vi "TOP VI-aim lab.vi"() -> ()   [LabVIEW 2014]
uses:
  <vilib>/Utility/miscctls.llb/LVPoint32TypeDef.ctl
  <vilib>/Utility/miscctls.llb/LVPositionTypeDef.ctl
panel:
  out "RECORD":bool
  in  "player name":string="player 1"
  out "element":T1(ring)
  out "seconds":dbl
  out "millisecond timer value 2":u32
  out "millisecond timer value":u32
  out "finish ?":bool
  out "Boolean":bool
  out "hit coord":T2
  in  "aim":bool
  in  "normal":bool
  in  "number of targets":i32=10
  in  "spacing limit":i32=5
  out "records":string[][](table)
  in  "New Game":bool
  in  "Quit":bool
  out "Game Image":picture
  # "true for aim mode"
  # "user discription:\npress New Game before run ensure parameters was set.\nchose mode with the lowest button;\npractice mode doesnt get records;\naim mode get records;\nrecords renew when vi restart;\nset name and parameter up to the \ndiscription;\npress New Game to change the number of targets & spacing limit;\n\n註記：\n右邊的picture大小可能與電腦螢幕大小有關，可用property調整為該使用者適當的螢幕大小，若是無法跑動，把play aim set target 跟generate target這兩個sub vi的cluster array重新創一次(不知道為啥有時會跑掉。目標有可能出現在視窗邊邊，須留意，畢竟有時敵人也只有露半個頭。"
  # "user pane"
  # "game pane"
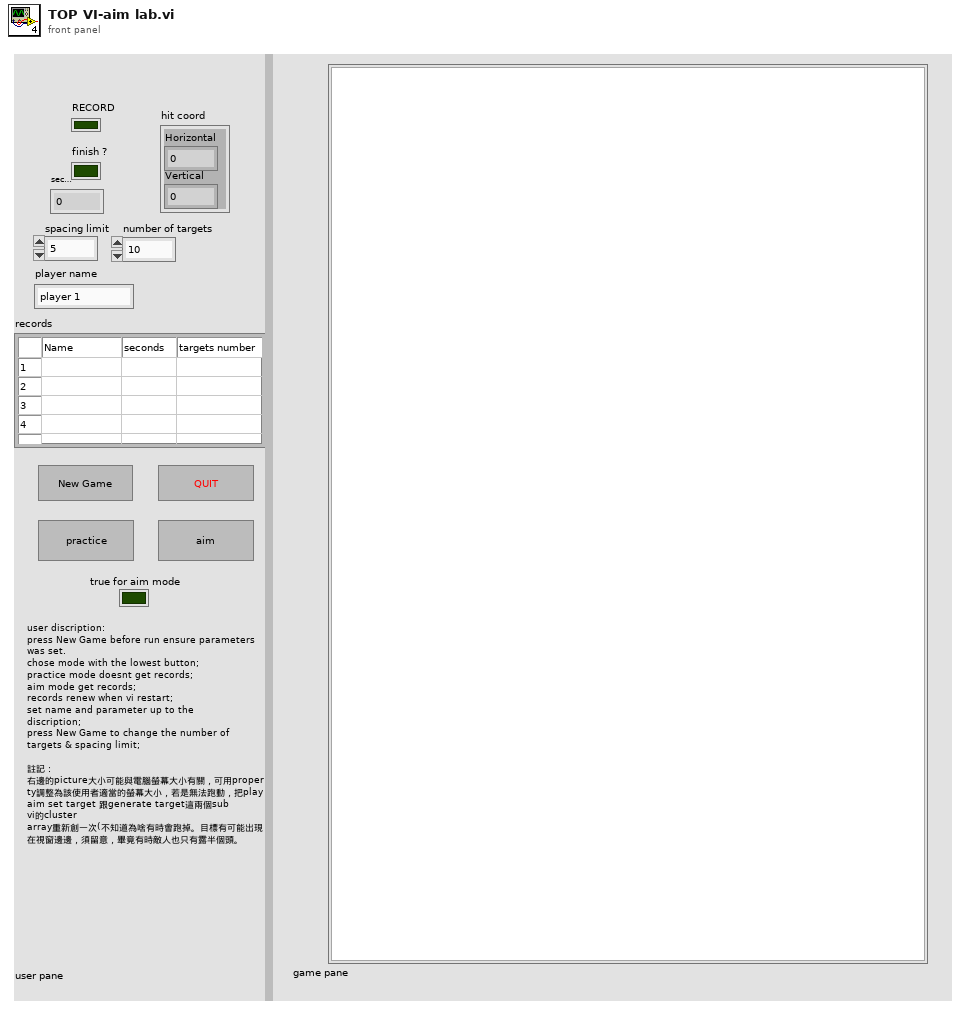
[diagram p1: front panel]
types:
  T1 = enum16{"waits function", "new game(reset)", "play normal", "play aim", "check hit", "quit", "draw target", "draw target for aim"}
  T2 = typedef "LVPoint32TypeDef.ctl" = cluster{"Horizontal":i32, "Vertical":i32}
  T3 = typedef "LVPositionTypeDef.ctl" = cluster{"Left":i32, "Top":i32}
  T4 = enum16{"nothing", "quit", "in play(normal or aim)"}
  T5 = enum16{"waits function", "new game(reset)", "play normal", "play aim", "check hit", "quit"}
  T6 = enum8{"Enabled", "Disabled", "Disabled and Grayed Out"}
  T7 = enum16{"waits function", "new game(reset)", "play normal", "play aim", "check hit", "quit", "draw target"}
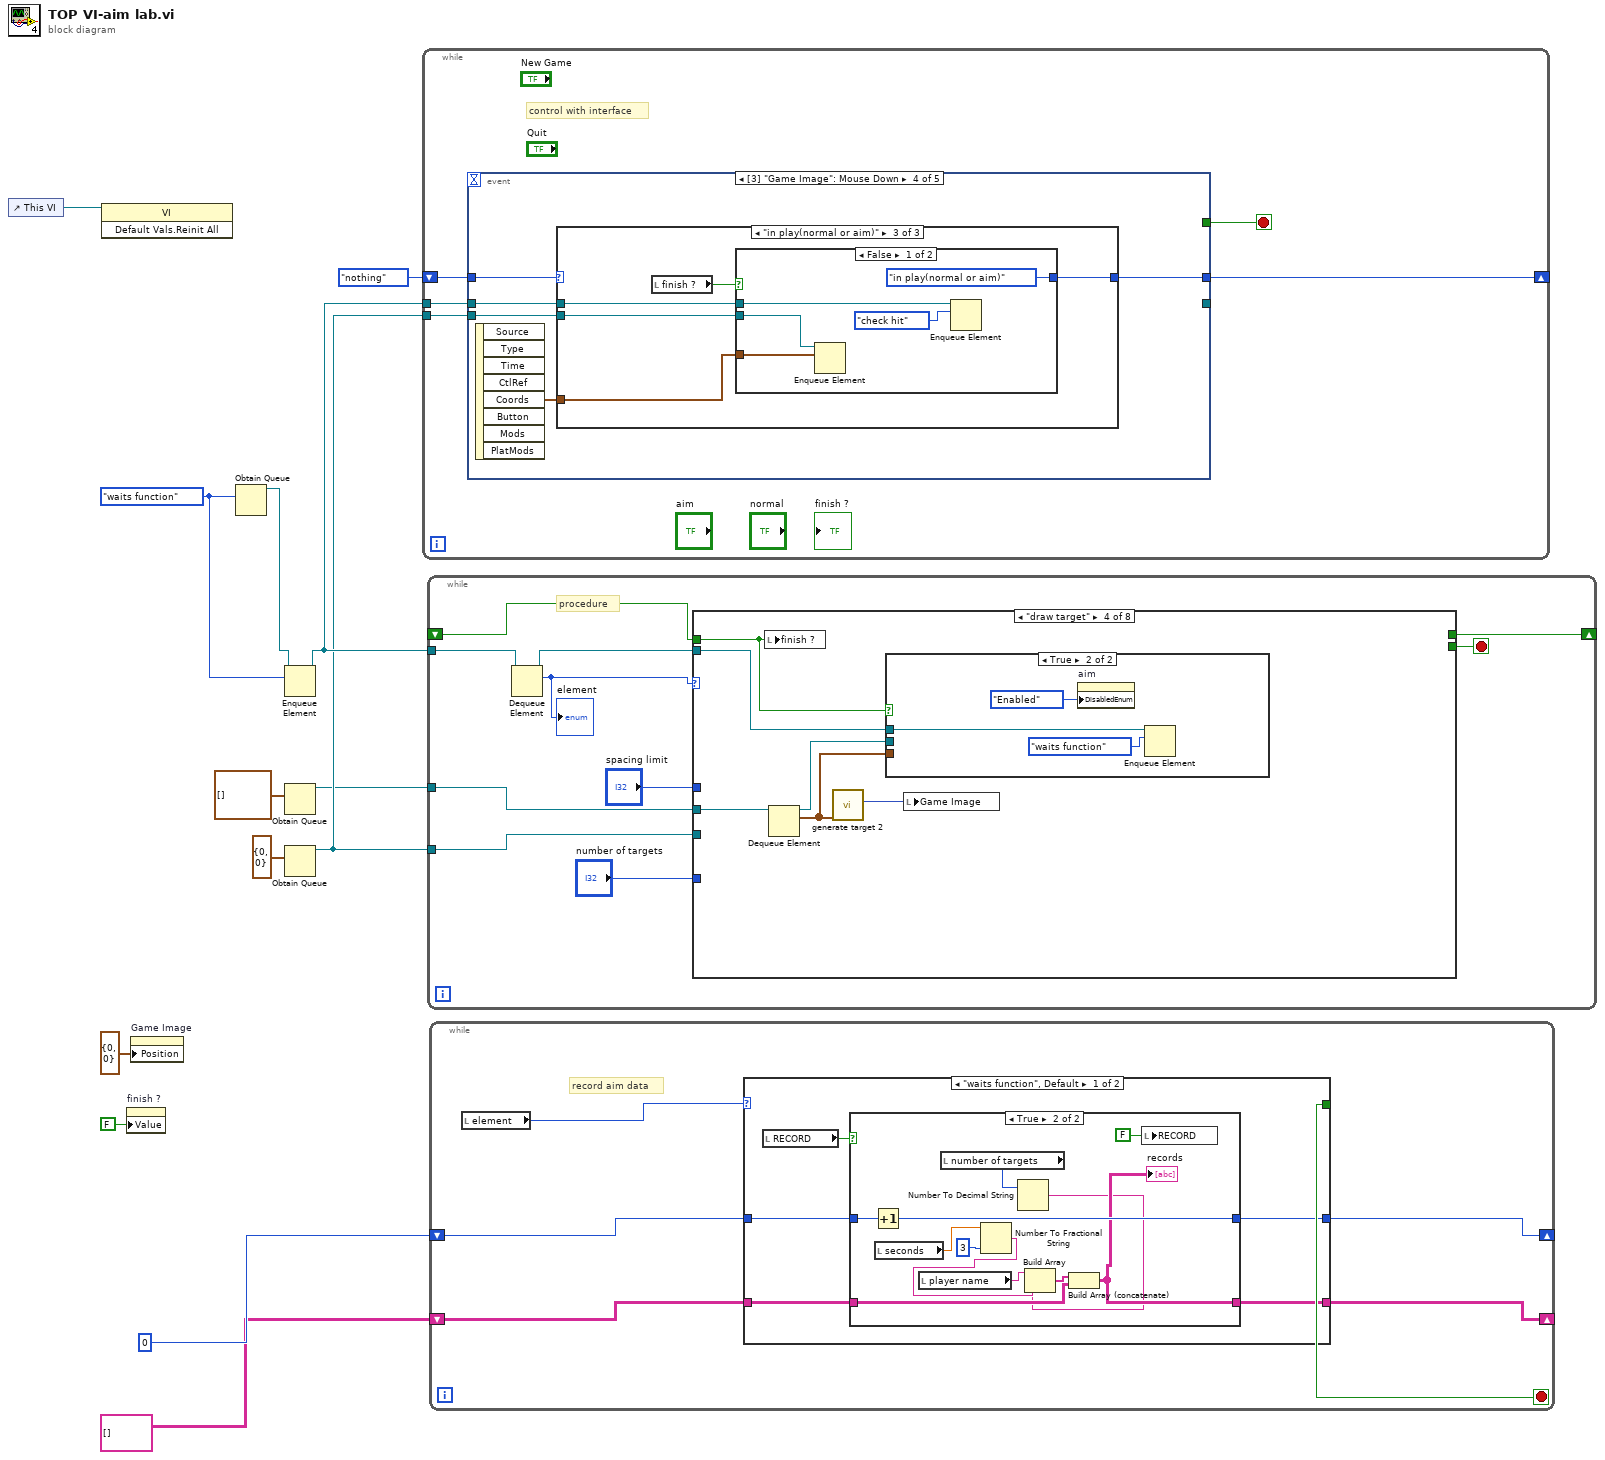
[diagram p0: block diagram]
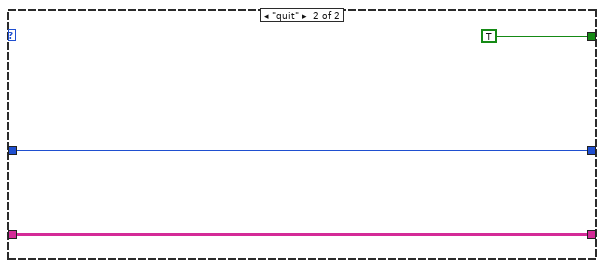
[diagram p3: hidden frame]
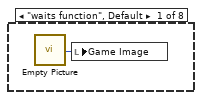
[diagram p4: hidden frame]
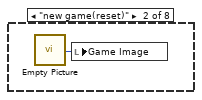
[diagram p5: hidden frame]
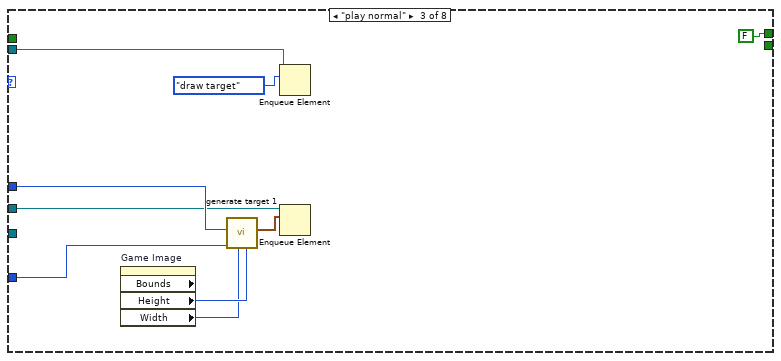
[diagram p6: hidden frame]
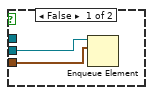
[diagram p7: hidden frame]
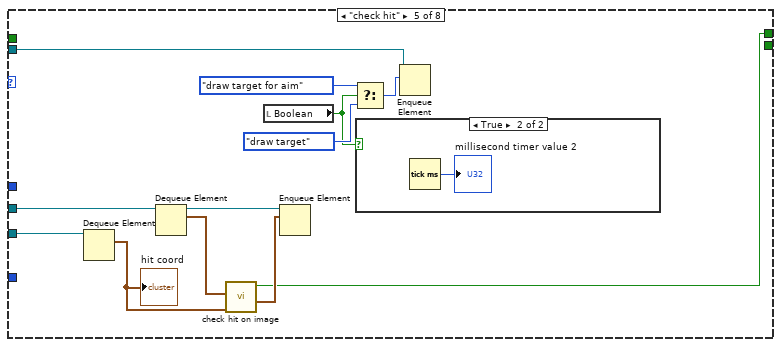
[diagram p8: hidden frame]
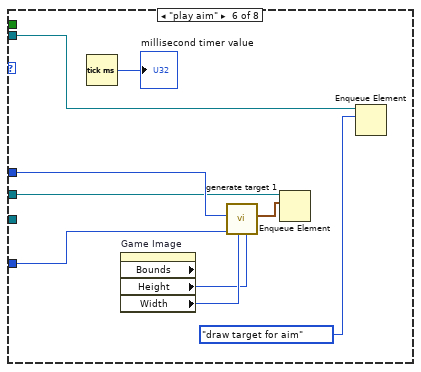
[diagram p10: hidden frame]
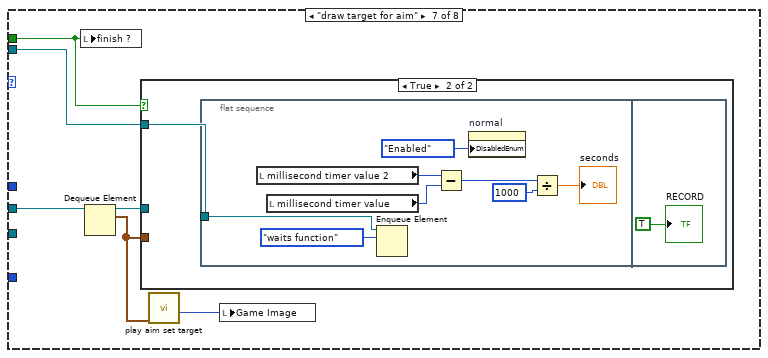
[diagram p11: hidden frame]
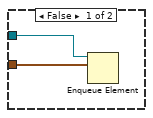
[diagram p12: hidden frame]
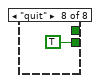
[diagram p13: hidden frame]
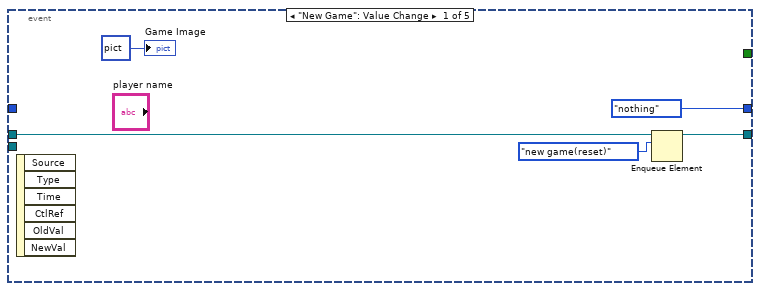
[diagram p14: hidden frame]
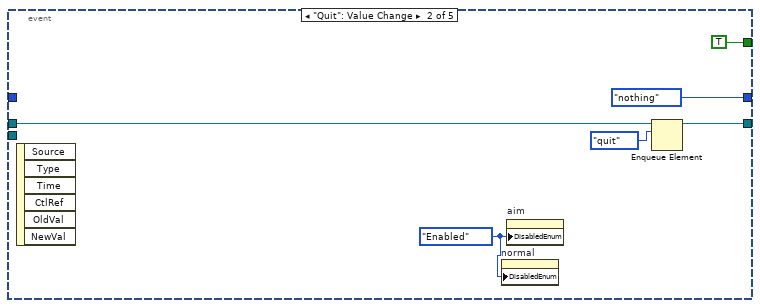
[diagram p15: hidden frame]
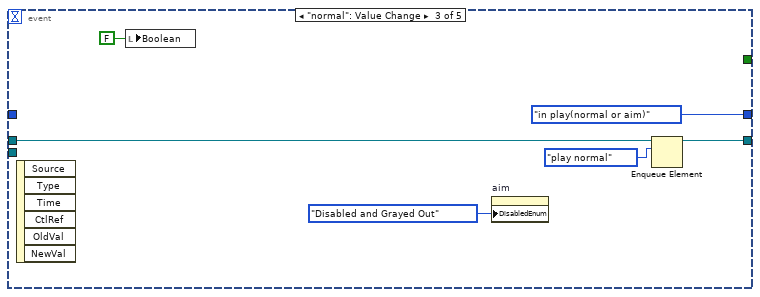
[diagram p16: hidden frame]
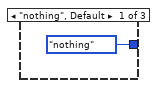
[diagram p17: hidden frame]
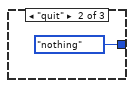
[diagram p18: hidden frame]
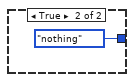
[diagram p19: hidden frame]
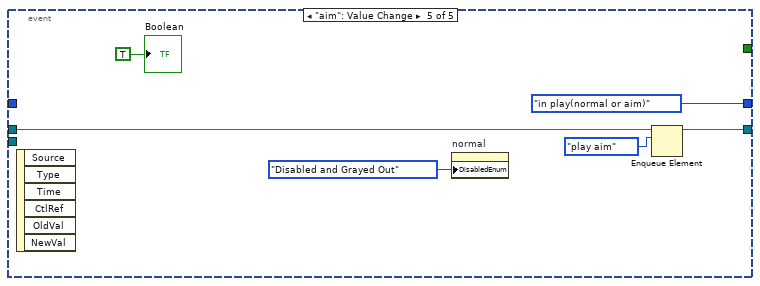
[diagram p20: hidden frame]
diagram:
  w13 = T1."waits function"
  n1 = control-ref of="This VI"() -> (w1:refnum<vi>)
  n2 = invoke class="VI" method="Default Vals.Reinit All"(reference=w1) -> ()  [unwired: 2 in, 3 out]
  n3 = property on="finish ?" class="Bool (strict)"("Value"=FALSE ("finish ?")) -> ()  [unwired: 2 in, 2 out]
  n4 = property on="Game Image" class="Pict"("Position"=T3 {"Left"=0, "Top"=0}) -> ()  [unwired: 2 in, 2 out]
  n5 = Obtain Queue(element data type=w13) -> (queue out=w12:refnum<queue>)  [unwired: 4 in, 2 out]
  n6 = Enqueue Element(queue=w12, element=w13) -> (queue out=w11:refnum<queue>)  [unwired: 2 in, 2 out]
  n7 = Obtain Queue(element data type=T2[] []) -> (queue out=w7:refnum<queue>)  [unwired: 4 in, 2 out]
  n8 = Obtain Queue(element data type=T2 {"Horizontal"=0, "Vertical"=0} ("Coords")) -> (queue out=w9:refnum<queue>)  [unwired: 4 in, 2 out]
  n9 = while {
    tunnel: w11 -> [w18]
    tunnel: w9 -> [w16]
    shift-right: [w14] -> _
    shift-left: T4."nothing" -> [w15]
    stop <- w17 stop-if-true
    # "control with interface"
    n10 = event shown="[3] \"Game Image\": Mouse Down" {
      selector: _ -> [_ _ _ _ _]
      dyn-events: _ -> [_ _ _ _ _]
      timeout: _ -> [_ _ _ _ _]
      tunnel: w18 -> [w23 w29 w35 w38 w59]
      tunnel: [w22 w28 w34 _ w58] -> _
      tunnel: [_ TRUE _ _ _] -> w17
      tunnel: w16 -> [_ _ _ w40 _]
      tunnel: w15 -> [_ _ _ w37 _]
      tunnel: [T4."nothing" T4."nothing" T4."in play(normal or aim)" w36 T4."in play(normal or aim)"] -> w14
      event "New Game": Value Change {
        n11 = event-data() -> ()  [unwired: 1 in, 6 out]
        n12 = Enqueue Element(queue=w23, element=T5."new game(reset)") -> (queue out=w22:refnum<queue>)  [unwired: 2 in, 2 out]
        "Game Image" <- picture bytes[15120] ("Game Image")
      }
      event "Quit": Value Change {
        w24 = T6."Enabled" ("Disabled")
        n13 = event-data() -> ()  [unwired: 1 in, 6 out]
        n14 = property on="normal" class="Bool"("DisabledEnum"=w24) -> ()  [unwired: 2 in, 2 out]
        n15 = property on="aim" class="Bool"("DisabledEnum"=w24) -> ()  [unwired: 2 in, 2 out]
        n16 = Enqueue Element(queue=w29, element=T5."quit") -> (queue out=w28:refnum<queue>)  [unwired: 2 in, 2 out]
      }
      event "normal": Value Change {
        n17 = event-data() -> ()  [unwired: 1 in, 6 out]
        n18 = local write "Boolean"(FALSE) -> ()
        n19 = property on="aim" class="Bool"("DisabledEnum"=T6."Disabled and Grayed Out" ("Disabled")) -> ()  [unwired: 2 in, 2 out]
        n20 = Enqueue Element(queue=w35, element=T5."play normal") -> (queue out=w34:refnum<queue>)  [unwired: 2 in, 2 out]
      }
      event "Game Image": Mouse Down {
        n21 = event-data() -> ("Coords"=w39:T2)  [unwired: 1 in, 7 out]
        n22 = case shown="\"in play(normal or aim)\"" w37 {
          tunnel: w40 -> [_ _ w47]
          tunnel: w39 -> [_ _ w46]
          tunnel: w38 -> [_ _ w45]
          tunnel: [T4."nothing" T4."nothing" w43] -> w36
          frame "nothing", Default {
          }
          frame "quit" {
          }
          frame "in play(normal or aim)" {
            n23 = local read "finish ?"() -> (w44:bool)
            n24 = case shown="False" w44 {
              tunnel: w47 -> [w52 _]
              tunnel: w46 -> [w51 _]
              tunnel: w45 -> [w49 _]
              tunnel: [T4."in play(normal or aim)" T4."nothing"] -> w43
              frame False {
                n25 = Enqueue Element(queue=w52, element=w51) -> ()  [unwired: 2 in, 3 out]
                n26 = Enqueue Element(queue=w49, element=T5."check hit") -> ()  [unwired: 2 in, 3 out]
              }
              frame True {
              }
            }
          }
        }
      }
      event "aim": Value Change {
        n27 = event-data() -> ()  [unwired: 1 in, 6 out]
        n28 = property on="normal" class="Bool"("DisabledEnum"=T6."Disabled and Grayed Out" ("Disabled")) -> ()  [unwired: 2 in, 2 out]
        n29 = Enqueue Element(queue=w59, element=T5."play aim") -> (queue out=w58:refnum<queue>)  [unwired: 2 in, 2 out]
        "Boolean" <- TRUE
      }
    }
  }
  n30 = while {
    tunnel: w11 -> [w69]
    tunnel: w9 -> [w64]
    tunnel: w7 -> [w65]
    shift-right: [w60] -> _
    shift-left: _ -> [w61]
    stop <- w68 stop-if-true
    # "procedure"
    n31 = Dequeue Element(queue=w69) -> (queue out=w62:refnum<queue>, element=w63:T1)  [unwired: 2 in, 2 out]
    "element" <- w63
    n32 = case shown="\"draw target\"" w63 {
      tunnel: [_ _ _ _ _ _ _ TRUE] -> w68
      tunnel: "spacing limit" -> [_ _ w78 _ _ w113 _ _]
      tunnel: "number of targets" -> [_ _ w77 _ _ w112 _ _]
      tunnel: w65 -> [_ _ w75 w85 w100 w108 w119 _]
      tunnel: w64 -> [_ _ _ _ w103 _ _ _]
      tunnel: w62 -> [_ _ w73 w84 w97 w107 w117 _]
      tunnel: [_ _ FALSE ("last target") _ w96 _ _ _] -> w60
      tunnel: w61 -> [_ _ _ w81 _ _ w114 _]
      frame "waits function", Default {
        n33 = call "Empty Picture"() -> ("empty picture"=w70:picture)
        n34 = local write "Game Image"(w70) -> ()
      }
      frame "new game(reset)" {
        n35 = call "Empty Picture"() -> ("empty picture"=w71:picture)
        n36 = local write "Game Image"(w71) -> ()
      }
      frame "play normal" {
        n37 = property on="Game Image" class="Pict" props=["Bounds", "Height", "Width"]() -> ("Height"=w80:u32, "Width"=w79:u32)  [unwired: 2 in, 3 out]
        n38 = call "generate target 1.vi"("PICTURE SIZE Y"=w80, "PICTURE SIZE X"=w79, "number of targets"=w77, "spacing limit"=w78) -> ("Array 2"=w76:cluster{"Numeric":i32, "Numeric 2":i32}[])  [unwired: 7 in]
        n39 = Enqueue Element(queue=w73, element=T7."draw target") -> ()  [unwired: 2 in, 3 out]
        n40 = Enqueue Element(queue=w75, element=w76) -> ()  [unwired: 2 in, 3 out]
      }
      frame "draw target" {
        n41 = local write "finish ?"(w81) -> ()
        n42 = Dequeue Element(queue=w85) -> (queue out=w83:refnum<queue>, element=w82:T2[])  [unwired: 2 in, 2 out]
        n43 = call "generate target 2.vi"("Array"=w82) -> ("2D Picture"=w86:picture)  [unwired: 10 in]
        n44 = case shown="True" w81 {
          tunnel: w84 -> [_ w90]
          tunnel: w83 -> [w88 _]
          tunnel: w82 -> [w87 _]
          frame False {
            n45 = Enqueue Element(queue=w88, element=w87) -> ()  [unwired: 2 in, 3 out]
          }
          frame True {
            n46 = property on="aim" class="Bool"("DisabledEnum"=T6."Enabled" ("Disabled")) -> ()  [unwired: 2 in, 2 out]
            n47 = Enqueue Element(queue=w90, element=T7."waits function") -> ()  [unwired: 2 in, 3 out]
          }
        }
        n48 = local write "Game Image"(w86) -> ()
      }
      frame "check hit" {
        n49 = Dequeue Element(queue=w103) -> (element=w102:T2)  [unwired: 2 in, 3 out]
        "hit coord" <- w102
        n50 = Dequeue Element(queue=w100) -> (queue out=w99:refnum<queue>, element=w98:T2[])  [unwired: 2 in, 2 out]
        n51 = call "check hit on image.vi"("Cluster"=w102, "Array"=w98) -> ("Array 2"=w101:cluster{"Numeric":i32, "Numeric 2":i32}[], "last target"=w96:bool)  [unwired: 8 in]
        n52 = local read "Boolean"() -> (w92:bool)
        n53 = Enqueue Element(queue=w99, element=w101) -> ()  [unwired: 2 in, 3 out]
        n54 = Select(t=T1."draw target for aim", s=w92, f=T7."draw target") -> (s? t:f=w93:T1)
        n55 = case shown="True" w92 {
          frame False {
          }
          frame True {
            n56 = Tick Count (ms)() -> (millisecond timer value=→"millisecond timer value 2":u32)
          }
        }
        n57 = Enqueue Element(queue=w97, element=w93) -> ()  [unwired: 2 in, 3 out]
      }
      frame "play aim" {
        n58 = Tick Count (ms)() -> (millisecond timer value=→"millisecond timer value":u32)
        n59 = property on="Game Image" class="Pict" props=["Bounds", "Height", "Width"]() -> ("Height"=w110:u32, "Width"=w111:u32)  [unwired: 2 in, 3 out]
        n60 = call "generate target 1.vi"("PICTURE SIZE Y"=w110, "PICTURE SIZE X"=w111, "number of targets"=w112, "spacing limit"=w113) -> ("Array 2"=w109:cluster{"Numeric":i32, "Numeric 2":i32}[])  [unwired: 7 in]
        n61 = Enqueue Element(queue=w108, element=w109) -> ()  [unwired: 2 in, 3 out]
        n62 = Enqueue Element(queue=w107, element=T1."draw target for aim") -> ()  [unwired: 2 in, 3 out]
      }
      frame "draw target for aim" {
        n63 = local write "finish ?"(w114) -> ()
        n64 = Dequeue Element(queue=w119) -> (queue out=w116:refnum<queue>, element=w115:T2[])  [unwired: 2 in, 2 out]
        n65 = case shown="True" w114 {
          tunnel: w117 -> [_ w122]
          tunnel: w116 -> [w121 _]
          tunnel: w115 -> [w120 _]
          frame False {
            n66 = Enqueue Element(queue=w121, element=w120) -> ()  [unwired: 2 in, 3 out]
          }
          frame True {
            n67 = flat-sequence {
              tunnel: w122 -> [w129]
              frame #0 {
                n68 = local read "millisecond timer value 2"() -> (w128:u32)
                n69 = local read "millisecond timer value"() -> (w127:u32)
                n70 = Enqueue Element(queue=w129, element=T7."waits function") -> ()  [unwired: 2 in, 3 out]
                n71 = Subtract(x=w128, y=w127) -> (x-y=w126:u32)
                n72 = property on="normal" class="Bool"("DisabledEnum"=T6."Enabled" ("Disabled")) -> ()  [unwired: 2 in, 2 out]
                n73 = Divide(x=w126, y=u32 1000) -> (x/y=→"seconds":dbl)
              }
              frame #1 {
                "RECORD" <- TRUE
              }
            }
          }
        }
        n74 = call "play aim set target.vi"("Array"=w115) -> ("2D Picture"=w118:picture)  [unwired: 10 in]
        n75 = local write "Game Image"(w118) -> ()
      }
      frame "quit" {
      }
    }
  }
  n76 = while {
    shift-right: [w133] -> _
    shift-left: string[][] [] -> [w136]
    shift-right: [w134] -> _
    shift-left: 0 -> [w135]
    stop <- w137 stop-if-true
    # "record aim data"
    n77 = local read "element"() -> (w138:T1)
    n78 = case shown="\"waits function\", Default" w138 {
      tunnel: [_ TRUE] -> w137
      tunnel: w136 -> [w141 w158]
      tunnel: w135 -> [w143 w159]
      tunnel: [w142 w159] -> w134
      tunnel: [w140 w158] -> w133
      frame "waits function", Default {
        n79 = local read "RECORD"() -> (w139:bool)
        n80 = case shown="True" w139 {
          tunnel: w143 -> [w145 w157]
          tunnel: [w145 w156] -> w142
          tunnel: w141 -> [w144 w154]
          tunnel: [w144 w148] -> w140
          frame False {
          }
          frame True {
            n81 = Increment(x=w157) -> (x+1=w156:i32)
            n82 = local read "seconds"() -> (w152:dbl)
            n83 = local read "player name"() -> (w150:string)
            n84 = local read "number of targets"() -> (w147:i32)
            n85 = Number To Fractional String(number=w152, precision (6)=i16 3) -> (F-format string=w149:string)  [unwired: 2 in]
            n86 = Number To Decimal String(number=w147) -> (decimal integer string=w146:string)  [unwired: 1 in]
            n87 = Build Array(w150, w149, w146) -> (w155:string[])
            n88 = Build Array (concatenate)(w155, w154) -> (w148:string[][])
            "records" <- w148
            n89 = local write "RECORD"(FALSE) -> ()
          }
        }
      }
      frame "quit" {
      }
    }
  }
